vi "LD2018_ブロック崩し_境界チェック.vi"(11 "Ball座標":cluster{dbl, dbl, dbl, dbl}) -> (3 "接触点":i32(ring) items=["なし", "上", "左", "右", "下"])   [LabVIEW 2016]
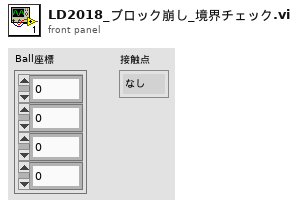
[diagram p1: front panel]
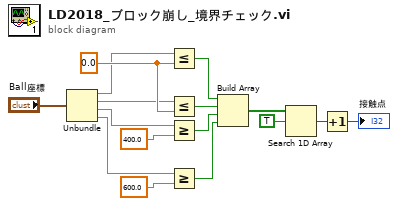
[diagram p0: block diagram]
diagram:
  w16 = 0.0 ("y")
  n1 = Unbundle("Ball座標") -> (w9:dbl, w1:dbl, w13:dbl, w11:dbl)
  n2 = Less Or Equal?(x=w9, y=w16) -> (x <= y?=w10:bool)
  n3 = Less Or Equal?(x=w1, y=w16) -> (x <= y?=w3:bool)
  n4 = Greater Or Equal?(x=w13, y=400.0) -> (x >= y?=w4:bool)
  n5 = Greater Or Equal?(x=w11, y=600.0) -> (x >= y?=w12:bool)
  n6 = Build Array(w10, w3, w4, w12) -> (w5:bool[])
  n7 = Search 1D Array(1D array=w5, element=TRUE ("要素")) -> (index of element=w7:i32)  [unwired: 1 in]
  n8 = Increment(x=w7) -> (x+1=→"接触点":i32)
